vi "ConcatTwoStrings_LV2009SP1.vi"(1 "String 2":string, 2 "String":string) -> (0 "String 3":string)   [LabVIEW 2009]
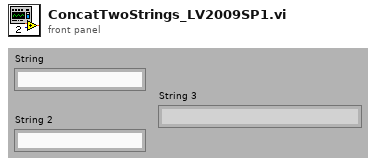
[diagram p1: front panel]
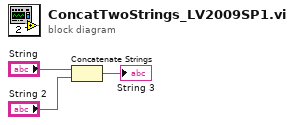
[diagram p0: block diagram]
diagram:
  n1 = Concatenate Strings("String", "String 2") -> (→"String 3":string)
